vi "One Camera.vi"() -> ()   [LabVIEW 2015]
uses:
  <vilib>/userdefined/High Color/IMAQdx.ctl
  Controls/Save picture camera.vi
  <vilib>/vision/driver/NI_Vision_Acquisition_Software.lvlib
panel:
  in  "布尔":bool
  in  "Session In":T1="cam2"
  in  "Path":path=path "C:/Users/T7610/Desktop/test" caption="Images Folder"
  in  "File Name":string
  out "Image Number":u32=99
  out "Frame Rate":dbl=4.987531172069826
  in  "Stop":bool
  out "Image":T2(plugin-control)
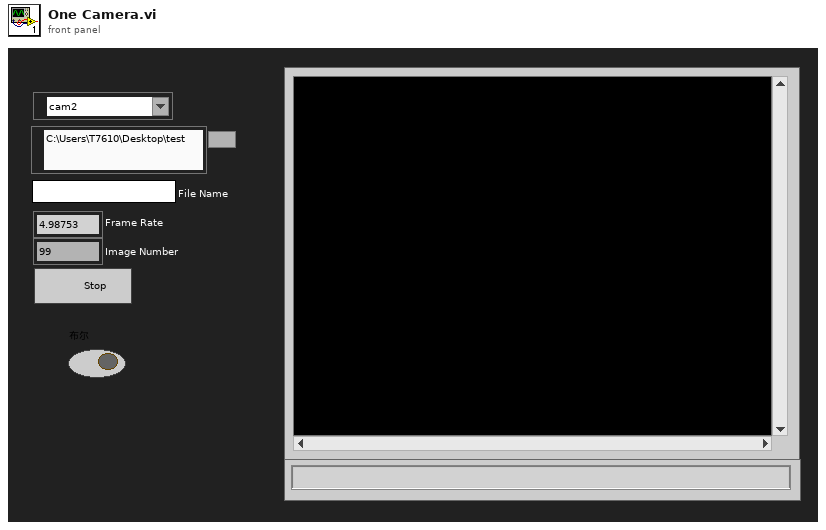
[diagram p1: front panel]
types:
  T1 = typedef "IMAQdx.ctl" = refnum<k21>
  T2 = typedef "IMAQ Image.ctl" = refnum<image>
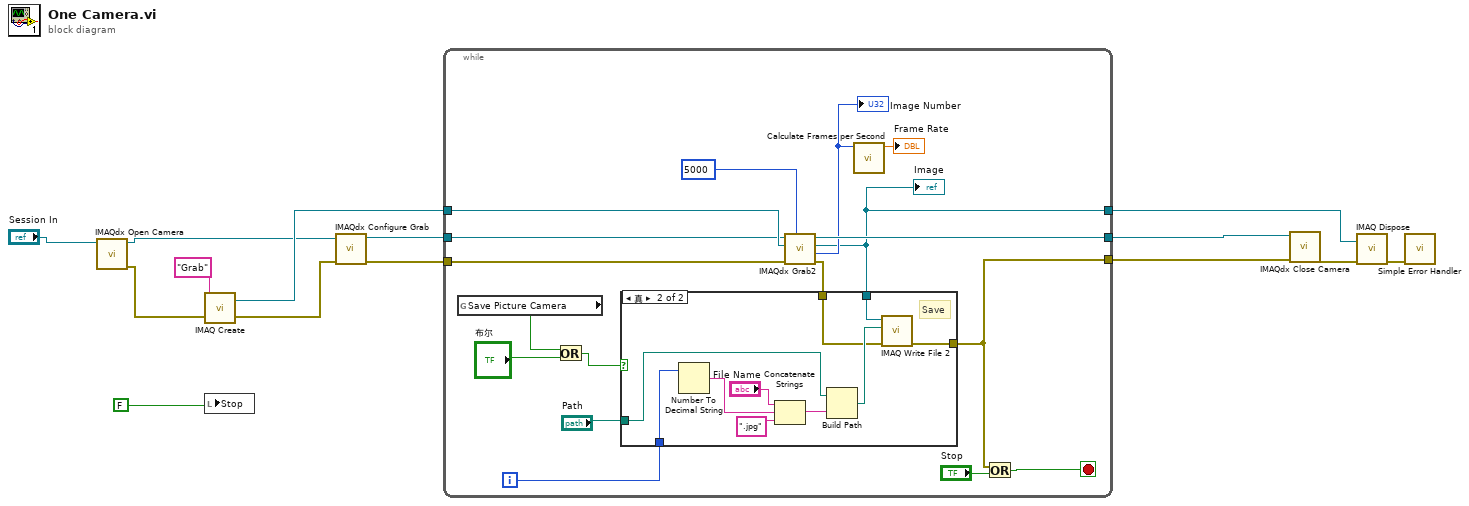
[diagram p0: block diagram]
diagram:
  n1 = call <vilib>:"IMAQdx Open Camera.vi"("Session In"="Session In") -> ("error out"=w9:errorcluster, "Session Out"=w8:T1)  [unwired: 9 in]
  n2 = call "IMAQ Create"("Image Name"="Grab", "error in (no error)"=w9) -> ("New Image"=w13:T2, "error out"=w2:errorcluster)  [unwired: 2 in, 1 out]
  n3 = local write "Stop"(FALSE ("Stop")) -> ()
  n4 = call <vilib>:"IMAQdx Configure Grab.vi"("error in"=w2, "Session In"=w8) -> ("error out"=w4:errorcluster, "Session Out"=w7:T1)  [unwired: 8 in]
  n5 = while {
    tunnel: [w28] -> w6
    tunnel: w13 -> [w29]
    tunnel: w4 -> [w24]
    tunnel: [w21] -> w12
    tunnel: w7 -> [w25]
    tunnel: [w19] -> w3
    i -> [w22]
    stop <- w31 stop-if-true
    n6 = global read "Save picture camera.vi" "Save Picture Camera"() -> (w17:bool)
    n7 = Or(x=w17, y="布尔") -> (x .or. y?=w15:bool)
    n8 = call <vilib>:"IMAQdx Grab2.vi"("Timeout (ms)"=5000, "error in"=w24, "Image In"=w29, "Session In"=w25) -> ("error out"=w20:errorcluster, "Buffer Number Out"=w26:u32, "Image Out"=w21:T2, "Session Out"=w28:T1)  [unwired: 4 in]
    "Image" <- w21
    "Image Number" <- w26
    n9 = case shown="真" w15 {
      tunnel: "Path" -> [_ w37]
      tunnel: w22 -> [_ w36]
      tunnel: w21 -> [_ w35]
      tunnel: w20 -> [w32 w34]
      tunnel: [w32 w33] -> w19
      frame False {
      }
      frame True {
        # "Save"
        n10 = Number To Decimal String(number=w36) -> (decimal integer string=w39:string)  [unwired: 1 in]
        n11 = Concatenate Strings("File Name", w39, ".jpg" ("字符串")) -> (w38:string)
        n12 = Build Path(base path=w37, name or relative path=w38) -> (appended path=w41:path)
        n13 = call-poly "IMAQ Write File 2"("error in (no error)"=w34, "File Path"=w41, "Image"=w35) -> ("error out"=w33:errorcluster)  [unwired: 7 in, 1 out]
      }
    }
    n14 = call <vilib>:"Calculate Frames per Second.vi"("Buffer Number"=w26) -> ("Acquired Frames/s"=→"Frame Rate":dbl)  [unwired: 2 in, 8 out]
    n15 = Or(x=w19, y="Stop") -> (x .or. y?=w31:bool)
  }
  n16 = call <vilib>:"IMAQdx Close Camera.vi"("error in"=w3, "Session In"=w6) -> ("error out"=w5:errorcluster)  [unwired: 9 in]
  n17 = call "IMAQ Dispose"("Image"=w12, "error in (no error)"=w5) -> ("error out"=w11:errorcluster)  [unwired: 1 in, 3 out]
  n18 = call <vilib>:"Simple Error Handler.vi"("error in (no error)"=w11) -> ()  [unwired: 1 in, 8 out]
